vi "Work_Condition.vi"() -> ()   [LabVIEW 2014]
panel:
  in  "工作条件":string[][](table)
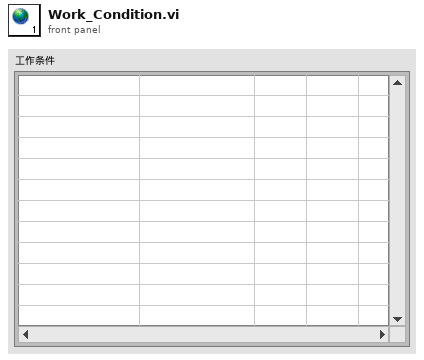
[diagram p1: front panel]
diagram:
